vi "send RT command.vi"(10 "comms in":T1, 11 "data":variant) -> (1 "timed out?":bool)   [LabVIEW 2018]
uses:
  type defs/comms loop data.ctl
  Chris VIs/Incident logger/Incident logger.lvclass
  <vilib>/Modbus/master/Modbus Master.lvclass
  <resource>/objmgr/ni.dex.rc
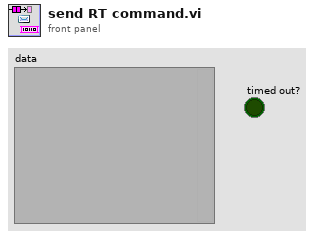
[diagram p1: front panel]
types:
  T1 = typedef "comms loop data.ctl" = cluster{"params":cluster{"commandStream":cluster{"reader name":string, "writer name":string, "stream buffer size":i32}, "errorStream":cluster{"reader name":string, "writer name":string, "stream buffer size":i32}, "RT IP address":string, "pulserControllerIP":string}, "vars":cluster{"commandStream":refnum<k21>, "Incident logger":refnum<class "Incident logger.lvclass">, "check error scheduled message":u32, "errorStream":refnum<k21>, "watchdogScheduleID":u32, "pulsator":cluster{"pulser connection":refnum<class "Modbus Master.lvclass">, "pulserConnected":bool, "pulsatorScheduleID":u32, "pulserRunning":bool}}}
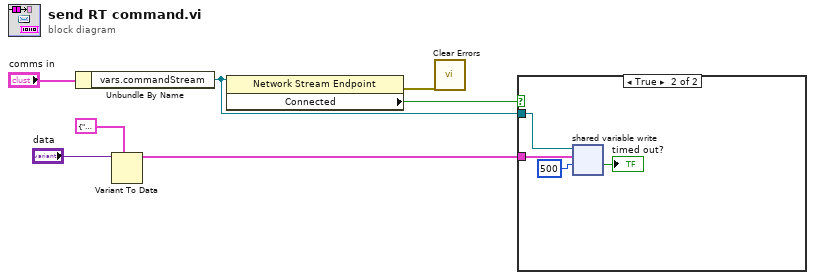
[diagram p0: block diagram]
diagram:
  n1 = Unbundle By Name("comms in") -> ("vars.commandStream"=w3:refnum<k21>)
  n2 = Variant To Data(type=cluster{"message":string, "data":variant} {"message"="", "data"=variant}, Variant="data") -> (data=w2:cluster{"message":string, "data":variant})  [unwired: 1 in, 1 out]
  n3 = property class="Network Stream Endpoint"(reference=w3) -> (error out=w1:errorcluster, "Connected"=w4:bool)  [unwired: 1 in, 1 out]
  n4 = call <vilib>:"Clear Errors.vi"("error in (no error)"=w1) -> ()  [unwired: 5 in, 2 out]
  n5 = case shown="True" w4 {
    tunnel: w3 -> [_ w11]
    tunnel: w2 -> [_ w10]
    frame False {
      # "add error handling here"
    }
    frame True {
      n6 = shared-variable-write(w11, w10, 500 ("timeout ms (-1)")) -> (→"timed out?":bool)  [unwired: 1 in, 2 out]
    }
  }
